vi "StrikerNormal.vi"(6 "atacando ao contrário?":bool=TRUE, 8 "IA Input":T6={"our_robots"=[], "enemy_robots"=[], "balls"=[], "geometry"={"line_width"=0, "field_length"=0, "field_width"=0, "boundary_width"=0, "referee_width"=0, "goal_width"=0, "goal_depth"=0, "goal_wall_width"=0, "center_circle_radius"=0, "defense_radius"=0, "defense_stretch"=0, "free_kick_from_defense_dist"=0, "penalty_spot_from_field_line_dist"=0, "penalty_line_from_spot_dist"=0}, "IA Judge"={"stage"="", "command"="", "our_goalie_id"=0.0, "enemy_goalie_id"=0.0, "command enum"=enum."Halt", "Time"=enum."Azul"}, "Received Timestamp"=timestamp(0 s since 1904-01-01), "Events"={"Touch"=FALSE, "Ball out"=FALSE, "id touch"=0.0, "Ball out of \nVision"=FALSE, "Ball inside \nGoalie area"=FALSE, "Robot not responding"=FALSE, "Robots responding status"=[1.0, 1.0, 1.0, 1.0, 1.0, 1.0], "Enemy Ball \nPossession"=FALSE, "Pass State"=FALSE, "id end of pass"=0.0, "Kick"=FALSE}}, 9 "balls":T4[](array[typedef])=[{"x"=-2165.869384765625, "y"=510.4085693359375, "timestamp"=timestamp(2082758857.4639893 s since 1904-01-01), "Vel_x"=0.0, "Vel_y"=0.0}], 10 "Field Size in":T5={"line_width"=10, "field_length"=6000, "field_width"=4000, "boundary_width"=250, "referee_width"=425, "goal_width"=700, "goal_depth"=180, "goal_wall_width"=20, "center_circle_radius"=500, "defense_radius"=500, "defense_stretch"=350, "free_kick_from_defense_dist"=700, "penalty_spot_from_field_line_dist"=450, "penalty_line_from_spot_dist"=350}, 11 "Robot in":T1={"id"=5, "function"=enum."Attacker", "x"=-1842.5054931640625, "y"=520.60986328125, "orientation"=-2.7555055618286133, "v_tangent"=0.0, "v_normal"=0.0, "v_ang"=0.0, "kick_x"=0.0, "kick_z"=0.0, "dribble"=FALSE, "Timestamp"=timestamp(2082758857.4639893 s since 1904-01-01), "dest_x"=0.0, "dest_y"=0.0, "dest_orientation"=0.0, "estimatives"={"est_v_tangent"=0.0, "est_v_normal"=0.0, "est_vx"=0.0, "est_vy"=0.0}, "dest_x_kick"=0.0, "dest_y_kick"=0.0, "Gap Coord"=[], "States"=enum."GoToTangent"}) -> (2 "Robot out":T1={"id"=5, "function"=enum."Attacker", "x"=-1842.5054931640625, "y"=520.60986328125, "orientation"=-2.7555055618286133, "v_tangent"=-0.08361641967936218, "v_normal"=-0.20513016702014014, "v_ang"=0.24456003022714357, "kick_x"=0.0, "kick_z"=0.0, "dribble"=FALSE, "Timestamp"=timestamp(2082758857.4639893 s since 1904-01-01), "dest_x"=0.0, "dest_y"=0.0, "dest_orientation"=0.0, "estimatives"={"est_v_tangent"=0.0, "est_v_normal"=0.0, "est_vx"=0.0, "est_vy"=0.0}, "dest_x_kick"=0.0, "dest_y_kick"=0.0, "Gap Coord"=[], "States"=enum."GoToTangent"})   [LabVIEW 2016]
uses:
  Core/AI Robot.ctl
  Functions Enum.ctl
  AttackerStates.ctl
  Core/AI Input.ctl
  Core/AI Ball.ctl
  Core/Field Size.ctl
  Core/AI Judge.ctl
  Command Enum.ctl
  Util/Events/Events.ctl
panel:
  in  "IDattacker":dbl
  in  "Yattacker":dbl
  in  "Xattacker":dbl
  out "States":T3
  out "sentido":dbl
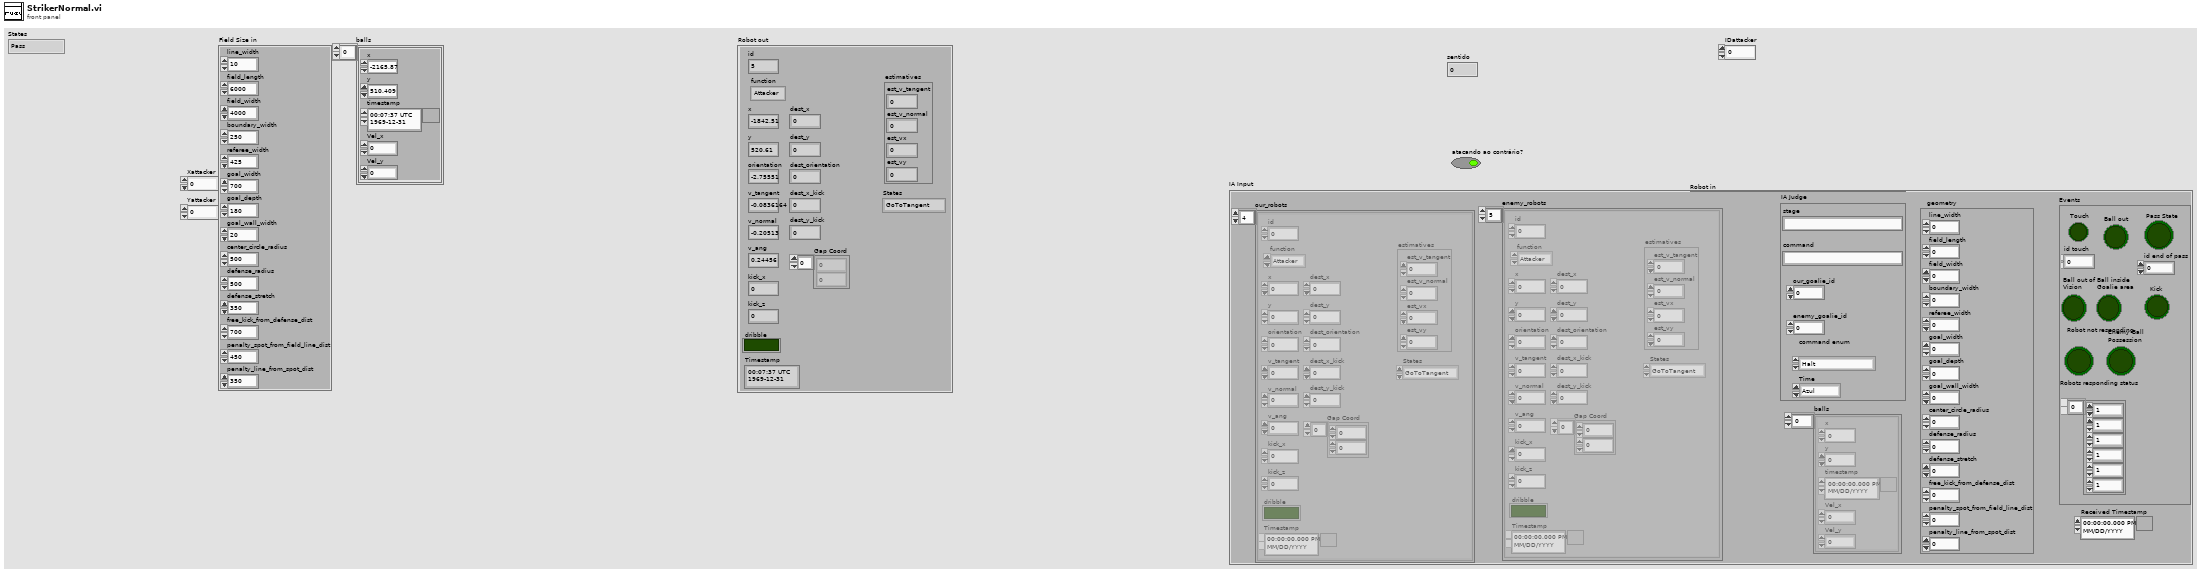
[diagram p1: front panel]
types:
  T1 = typedef "AI Robot.ctl" = cluster{"id":u32, "function":T2, "x":dbl, "y":dbl, "orientation":dbl, "v_tangent":dbl, "v_normal":dbl, "v_ang":dbl, "kick_x":dbl, "kick_z":dbl, "dribble":bool, "Timestamp":timestamp, "dest_x":dbl, "dest_y":dbl, "dest_orientation":dbl, "estimatives":cluster{"est_v_tangent":dbl, "est_v_normal":dbl, "est_vx":dbl, "est_vy":dbl}, "dest_x_kick":dbl, "dest_y_kick":dbl, "Gap Coord":dbl[], "States":T3}
  T2 = typedef "Functions Enum.ctl" = enum16{"Attacker", "Goalie", "Defender", "Striker", "Goto 0", "Dummy", "Kicker", "ZigZag"}
  T3 = typedef "AttackerStates.ctl" = enum16{"Pass", "GoToTangent", "BallGetting", "GoToKick", ""}
  T4 = typedef "AI Ball.ctl" = cluster{"x":dbl, "y":dbl, "timestamp":timestamp, "Vel_x":dbl, "Vel_y":dbl}
  T5 = typedef "Field Size.ctl" = cluster{"line_width":u32, "field_length":u32, "field_width":u32, "boundary_width":u32, "referee_width":u32, "goal_width":u32, "goal_depth":u32, "goal_wall_width":u32, "center_circle_radius":u32, "defense_radius":u32, "defense_stretch":u32, "free_kick_from_defense_dist":u32, "penalty_spot_from_field_line_dist":u32, "penalty_line_from_spot_dist":u32}
  T6 = typedef "AI Input.ctl" = cluster{"our_robots":T1[], "enemy_robots":T1[], "balls":T4[], "geometry":T5, "IA Judge":T7, "Received Timestamp":timestamp, "Events":T9}
  T7 = typedef "AI Judge.ctl" = cluster{"stage":string, "command":string, "our_goalie_id":dbl, "enemy_goalie_id":dbl, "command enum":T8, "Time":enum16{"Azul", "Amarelo"}}
  T8 = typedef "Command Enum.ctl" = enum16{"Halt", "Stop", "Force Start", "PKA Normal Start", "Prepare Kickoff Ally", "PKE Normal Start", "Prepare Kickoff Enemy", "Prepare Penalty Ally", "PPA Normal Start", "Prepare Penalty Enemy", "PPE Normal Start", "Direct Free Enemy", "Direct Free Ally", "Indirect Free Enemy", "Indirect Free Ally", "Timeout Enemy", "Timeout Ally", "Goal Enemy", "Goal Ally", "Ball Placement Enemy", "Ball Placement Ally", "Normal Half Time", "Extra Time Break", "Extra Half Time", "None"}
  T9 = typedef "Events.ctl" = cluster{"Touch":bool, "Ball out":bool, "id touch":dbl, "Ball out of \nVision":bool, "Ball inside \nGoalie area":bool, "Robot not responding":bool, "Robots responding status":dbl[], "Enemy Ball \nPossession":bool, "Pass State":bool, "id end of pass":dbl, "Kick":bool}
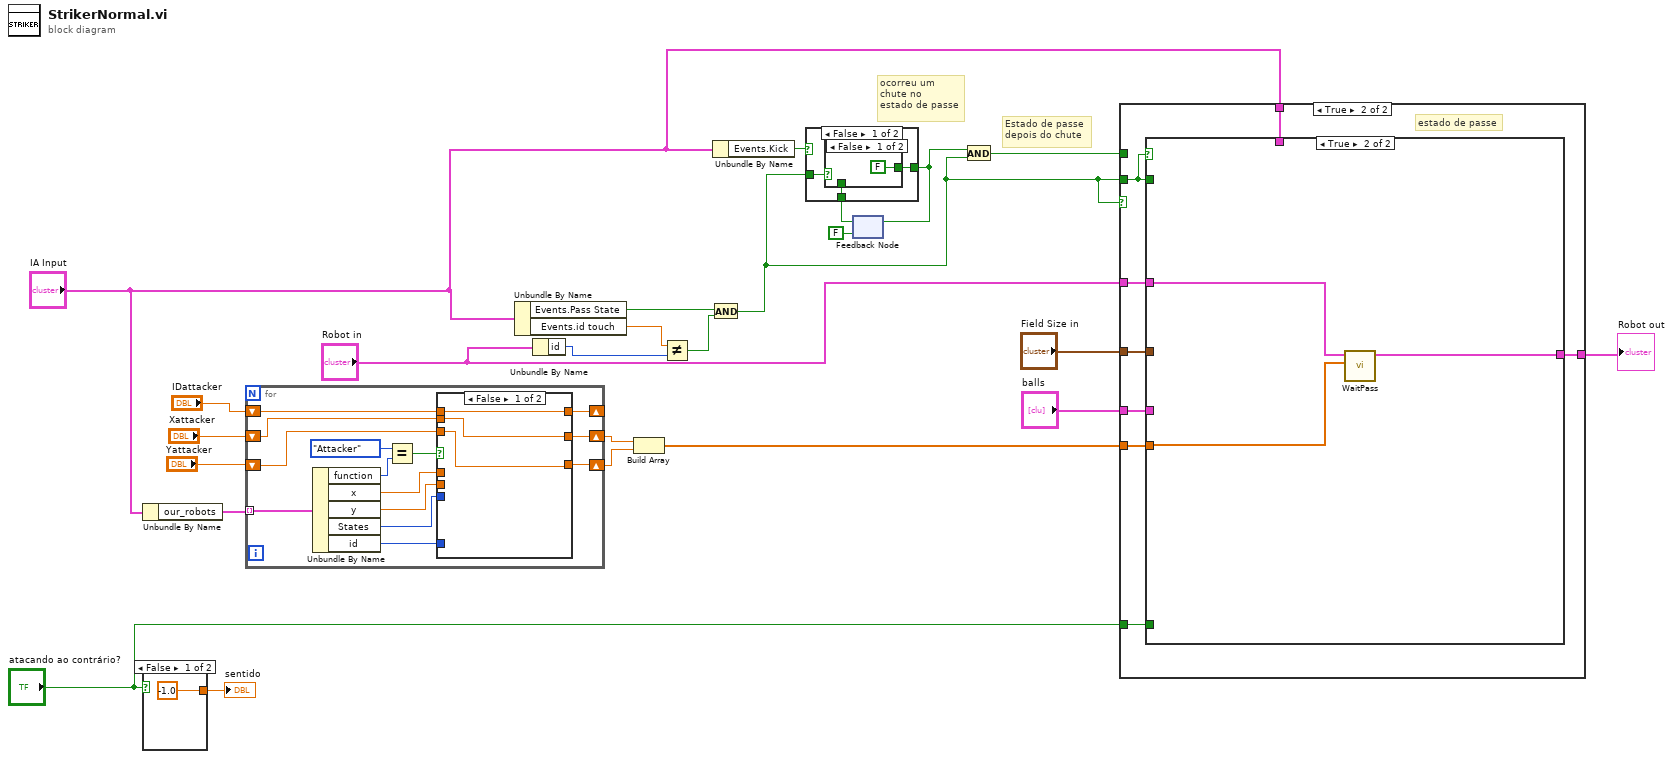
[diagram p0: block diagram]
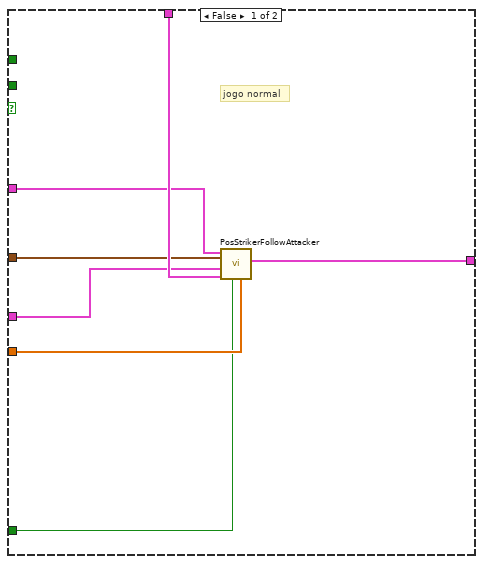
[diagram p2: hidden frame]
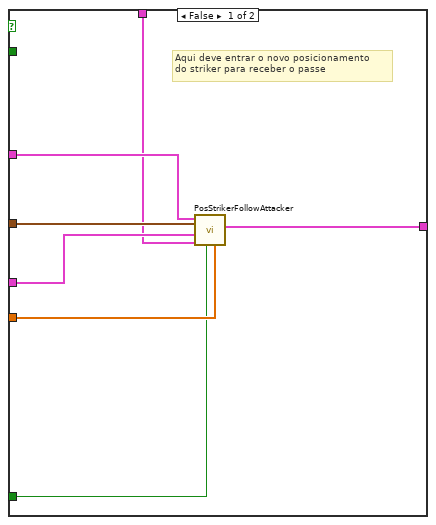
[diagram p3: hidden frame]
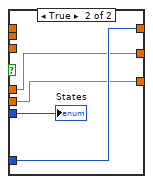
[diagram p4: hidden frame]
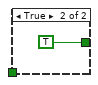
[diagram p6: hidden frame]
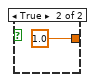
[diagram p7: hidden frame]
diagram:
  # "ocorreu um \nchute no\nestado de passe"
  # "Estado de passe\ndepois do chute"
  n1 = Unbundle By Name("IA Input") -> ("our_robots"=w17:T1[])
  n2 = case shown="False" "atacando ao contrário?" {
    tunnel: [-1.0 1.0] -> w24
    frame False {
    }
    frame True {
    }
  }
  "sentido" <- w24
  n3 = for {
    tunnel: w17 -> [w35] mode=indexing
    shift-right: [w31] -> w13
    shift-left: "Xattacker" -> [w29]
    shift-right: [w30] -> w12
    shift-left: "Yattacker" -> [w28]
    shift-right: [w32] -> _
    shift-left: "IDattacker" -> [w27]
    n4 = Unbundle By Name(w35) -> ("function"=w40:T2, "x"=w37:dbl, "y"=w36:dbl, "States"=w34:T3, "id"=w33:u32)
    n5 = Equal?(x=Functions_Enum."Attacker", y=w40) -> (x = y?=w38:bool)
    n6 = case shown="False" w38 {
      tunnel: w37 -> [_ w45]
      tunnel: w36 -> [_ w44]
      tunnel: w34 -> [_ w47]
      tunnel: w33 -> [_ w46]
      tunnel: [w41 w46] -> w32
      tunnel: [w43 w45] -> w31
      tunnel: [w42 w44] -> w30
      tunnel: w29 -> [w43 _]
      tunnel: w28 -> [w42 _]
      tunnel: w27 -> [w41 _]
      frame False {
      }
      frame True {
        "States" <- w47
      }
    }
  }
  n7 = Unbundle By Name("IA Input") -> ("Events.Pass State"=w18:bool, "Events.id touch"=w3:dbl)
  n8 = Unbundle By Name("Robot in") -> ("id"=w1:u32)
  n9 = Build Array(w13, w12) -> (w11:dbl[])
  n10 = Not Equal?(x=w3, y=w1) -> (x != y?=w4:bool)
  n11 = And(x=w18, y=w4) -> (x .and. y?=w5:bool)
  n12 = Unbundle By Name("IA Input") -> ("Events.Kick"=w23:bool)
  n13 = feedback #1(FALSE) -> (w21:bool)
  n14 = case shown="False" w23 {
    tunnel: [w49 TRUE] -> w22
    tunnel: w21 -> [w48 _]
    tunnel: w5 -> [w50 _]
    frame False {
      n15 = case shown="False" w50 {
        tunnel: [FALSE w52] -> w49
        tunnel: w48 -> [_ w52]
        frame False {
        }
        frame True {
        }
      }
    }
    frame True {
    }
  }
  n16 = feedback-in #1(w22) -> ()
  n17 = And(x=w22, y=w5) -> (x .and. y?=w19:bool)
  n18 = case shown="True" w5 {
    tunnel: w19 -> [_ _]
    tunnel: w5 -> [_ w61]
    tunnel: "Robot in" -> [w59 w68]
    tunnel: w11 -> [w56 w67]
    tunnel: "atacando ao contrário?" -> [w55 w66]
    tunnel: "Field Size in" -> [w58 w65]
    tunnel: "balls" -> [w57 w64]
    tunnel: "IA Input" -> [w60 w63]
    tunnel: [w54 w62] -> w6
    frame False {
      # "jogo normal"
      n19 = call "PosStrikerFollowAttacker.vi"("Pos Attacker"=w56, "atacando ao contrário?"=w55, "IA Input"=w60, "balls"=w57, "Field Size in"=w58, "Robot in"=w59) -> ("Robot out"=w54:T1)  [unwired: 5 in]
    }
    frame True {
      # "estado de passe"
      n20 = case shown="True" w61 {
        tunnel: w61 -> [_ _]
        tunnel: w68 -> [w73 w78]
        tunnel: w67 -> [w75 w77]
        tunnel: [w69 w76] -> w62
        tunnel: w66 -> [w74 _]
        tunnel: w65 -> [w72 _]
        tunnel: w64 -> [w71 _]
        tunnel: w63 -> [w70 _]
        frame False {
          # "Aqui deve entrar o novo posicionamento\ndo striker para receber o passe"
          n21 = call "PosStrikerFollowAttacker.vi"("Pos Attacker"=w75, "atacando ao contrário?"=w74, "IA Input"=w70, "balls"=w71, "Field Size in"=w72, "Robot in"=w73) -> ("Robot out"=w69:T1)  [unwired: 5 in]
        }
        frame True {
          n22 = call "WaitPass.vi"("Target"=w77, "Robot in"=w78) -> ("Robot out"=w76:T1)  [unwired: 9 in]
        }
      }
    }
  }
  "Robot out" <- w6
